vi "Drive.vi"(5 "SwitchDir":bool, 7 "Slow?":bool, 10 "Drive R":dbl, 11 "Drive L":dbl) -> ()   [LabVIEW 2016]
uses:
  <vilib>/Rock Robotics/WPI/SafetyOutput/WPI_SafetyOutputConfigMenu.ctl
panel:
  in  "LT":dbl format="%#_13g"
  in  "RT":dbl format="%#_13g"
  in  "Joystick 1":dbl=0.05511811023622047 format="%#_13g"
  out "Right":dbl=-0.05511811023622047 format="%#_13g"
  out "Left":dbl=0.05511811023622047 format="%#_13g"
  in  "Drive Reduction":dbl=0.4 format="%#_13g"
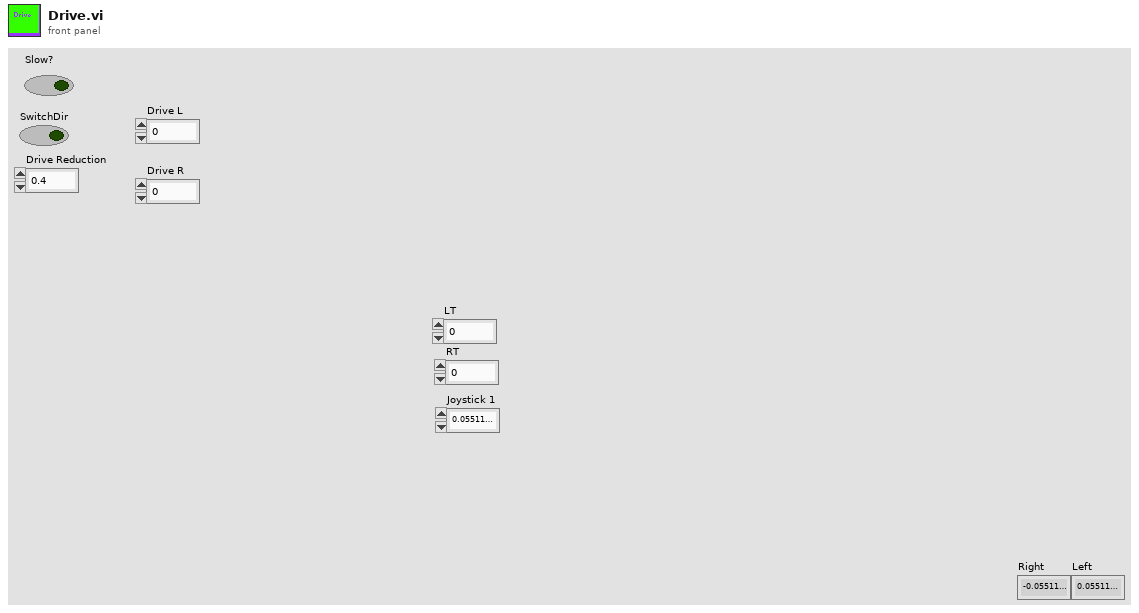
[diagram p1: front panel]
types:
  T1 = typedef "WPI_SafetyOutputConfigMenu.ctl" = enum16{"Enable", "Disable"}
  T2 = typedef "WPI_MotorControlDeviceRef.ctl" = cluster{"DeviceStatus":errorcluster, "Type":T3, "PWM":cluster{"PWM Channel":T4, "DeadBand":T5}, "CAN":cluster{"Device Number":u8, "SetOutput VI Ref":variant, "GetOutput VI Ref":variant, "Enable VI Ref":variant, "Disable VI Ref":variant, "Data":variant}, "Invert":bool}
  T3 = typedef "WPI_MotorControlType.ctl" = enum16{"PWM", "CAN"}
  T4 = typedef "FPGA_DIOPWMChannel.ctl" = enum8{"PWM 0", "PWM 1", "PWM 2", "PWM 3", "PWM 4", "PWM 5", "PWM 6", "PWM 7", "PWM 8", "PWM 9", "PWM MXP 0", "PWM MXP 1", "PWM MXP 2", "PWM MXP 3", "PWM MXP 4", "PWM MXP 5", "PWM MXP 6", "PWM MXP 7", "PWM MXP 8", "PWM MXP 9", "Invalid"}
  T5 = typedef "WPI_PWMDeadband.ctl" = cluster{"Name":string, "maxPositivePwm":i32, "minPositivePwm":i32, "centerPwm":i32, "maxNegativePwm":i32, "minNegativePwm":i32, "angularRange":u16}
  T6 = typedef "WPI_CANTalonSRX_GlobalStatus.ctl" = cluster{"Applied Throttle":dbl, "Module Enabled":bool, "CAN Error":errorcluster, "Closed Loop Error":dbl, "Forward Limit Switch Closed":bool, "Reverse Limit Switch Closed":bool, "Sensor Position":dbl, "Sensor Velocity":dbl, "Current":dbl, "Sticky Fault - Over Temp":bool, "Sticky Fault - Under Voltage":bool, "Sticky Fault - Forward Limit":bool, "Sticky Fault - Reverse Limit":bool, "Sticky Fault - Forward Soft Limit":bool, "Sticky Fault - Reverse Soft Limit":bool, "Brake is Enabled":bool, "Encoder Position":dbl, "Encoder Velocity":dbl, "Encoder Index Count":dbl, "Encoder A Pin State":bool, "Encoder B Pin State":bool, "Encoder Index Pin State":bool, "Analog In":dbl, "Analog In Velocity":dbl, "Temperature (C)":dbl, "Battery Voltage":dbl, "Control 5 Is Supported":bool, "Current Profile Slot Select":dbl, "Pos Div 8":bool, "Vel Div 4":bool, "Pulse Width Position":i32, "Pulse Width Velocity":i32, "Pulse Width Rise To Rise (us)":i32, "Pulse Width Rise To Fall (us)":i32, "Mot Prof Active Is Under Run":bool, "Mot Prof Active Has Under Run":bool, "Mot Prof Active Is Last":bool, "Mot Prof Active Velocity Only":bool, "Mot Prof Active Is Valid":bool, "Mot Prof Buffer Is Full":bool, "Mot Prof Active Profile Slot Select":i32, "Mot Prof NextID":i32, "Mot Prof Count":i32, "Mot Prof Active Velocity":dbl, "Mot Prof Active Position":dbl, "Mot Prof Output Enable":i32}
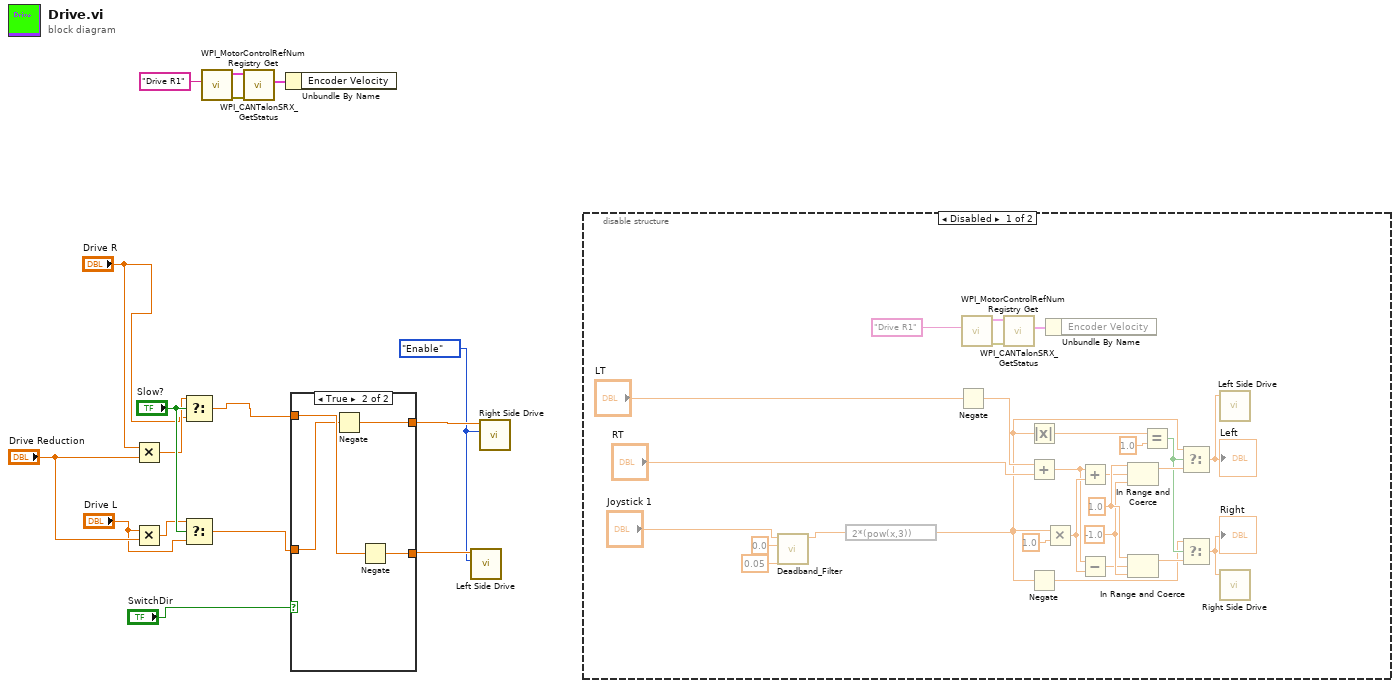
[diagram p0: block diagram]
diagram:
  w1 = WPI_SafetyOutputConfigMenu."Enable" ("mode")
  n1 = Multiply(x="Drive R", y="Drive Reduction") -> (x*y=w8:dbl)
  n2 = Multiply(x="Drive L", y="Drive Reduction") -> (x*y=w6:dbl)
  n3 = Select(t=w8, s="Slow?", f="Drive R") -> (s? t:f=w4:dbl)
  n4 = Select(t=w6, s="Slow?", f="Drive L") -> (s? t:f=w11:dbl)
  n5 = call <vilib>:"WPI_MotorControlRefNum Registry Get.vi"("refnum name"="Drive R1") -> ("error out"=w15:errorcluster, "MotorControlDevRef"=w16:T2)  [unwired: 9 in]
  n6 = call <vilib>:"WPI_CANTalonSRX_GetStatus.vi"("error in (no error)"=w15, "CAN Talon SRX Ref"=w16) -> ("Talon SRX Status"=w14:T6)  [unwired: 7 in, 2 out]
  n7 = Unbundle By Name(w14) -> ()  [unwired: 1 out]
  n8 = case shown="True" "SwitchDir" {
    tunnel: [w18 w20] -> w3
    tunnel: w4 -> [w18 w22]
    tunnel: [w17 w19] -> w2
    tunnel: w11 -> [w17 w21]
    frame False {
    }
    frame True {
      n9 = Negate(x=w21) -> (-x=w20:dbl)
      n10 = Negate(x=w22) -> (-x=w19:dbl)
    }
  }
  n11 = call "Left Side Drive.vi"("mode"=w1, "Effort"=w2) -> ()  [unwired: 10 in]
  n12 = call "Right Side Drive.vi"("mode"=w1, "Effort"=w3) -> ()  [unwired: 10 in]
  n13 = disable-structure shown="Disabled" {
    frame Disabled {
      w44 = -1.0 ("Numeric 4")
      w45 = 1.0 ("Numeric 4")
      n14 = call "Deadband_Filter.vi"("Range"=0.05, "Target"=0.0, "Joystick Input"="Joystick 1") -> ("Output"=w24:dbl)  [unwired: 8 in]
      n15 = expression code="2*(pow(x,3))"(w24) -> (w23:dbl)
      n16 = Negate(x="LT") -> (-x=w43:dbl)
      n17 = call <vilib>:"WPI_MotorControlRefNum Registry Get.vi"("refnum name"="Drive R1") -> ("error out"=w48:errorcluster, "MotorControlDevRef"=w49:T2)  [unwired: 9 in]
      n18 = call <vilib>:"WPI_CANTalonSRX_GetStatus.vi"("error in (no error)"=w48, "CAN Talon SRX Ref"=w49) -> ("Talon SRX Status"=w47:T6)  [unwired: 7 in, 2 out]
      n19 = Absolute Value(x=w23) -> (abs(x)=w37:dbl)
      n20 = Add(x=w43, y="RT") -> (x+y=w40:dbl)
      n21 = Negate(x=w23) -> (-x=w32:dbl)
      n22 = Multiply(x=w23, y=1.0) -> (x*y=w41:dbl)
      n23 = Unbundle By Name(w47) -> ()  [unwired: 1 out]
      n24 = Add(x=w40, y=w41) -> (x+y=w38:dbl)
      n25 = Subtract(x=w40, y=w41) -> (x-y=w39:dbl)
      n26 = In Range and Coerce(upper limit=w45, x=w38, lower limit=w44) -> (coerced(x)=w35:dbl)  [unwired: 1 out]
      n27 = In Range and Coerce(upper limit=w45, x=w39, lower limit=w44) -> (coerced(x)=w34:dbl)  [unwired: 1 out]
      n28 = Equal?(x=w37, y=1.0) -> (x = y?=w33:bool)
      n29 = Select(t=w23, s=w33, f=w35) -> (s? t:f=w29:dbl)
      "Left" <- w29
      n30 = Select(t=w32, s=w33, f=w34) -> (s? t:f=w28:dbl)
      "Right" <- w28
      n31 = call "Left Side Drive.vi"("Effort"=w29) -> ()  [unwired: 11 in]
      n32 = call "Right Side Drive.vi"("Effort"=w28) -> ()  [unwired: 11 in]
    }
    frame Enabled {
    }
  }
